vi "Driving.vi"(11 "input cluster":T2) -> (3 "Motor Info Cluster":T1)   [LabVIEW 2015]
uses:
  Joystick/ControlsToCommands.ctl
  References/Refnums.vi
panel:
  in  "Motor Values and Errors":T1
  out "Boolean":bool
  in  "valS":bool
  in  "PWM 5":dbl min=-1.0 max=1.0 step=1.0
  in  "PWM 4":dbl min=-1.0 max=1.0 step=1.0
  in  "PWM 3":dbl min=-1.0 max=1.0 step=1.0
  in  "PWM 2":dbl min=-1.0 max=1.0 step=1.0
  in  "PWM 1":dbl min=-1.0 max=1.0 step=1.0
  in  "PWM 0":dbl min=-1.0 max=1.0 step=1.0
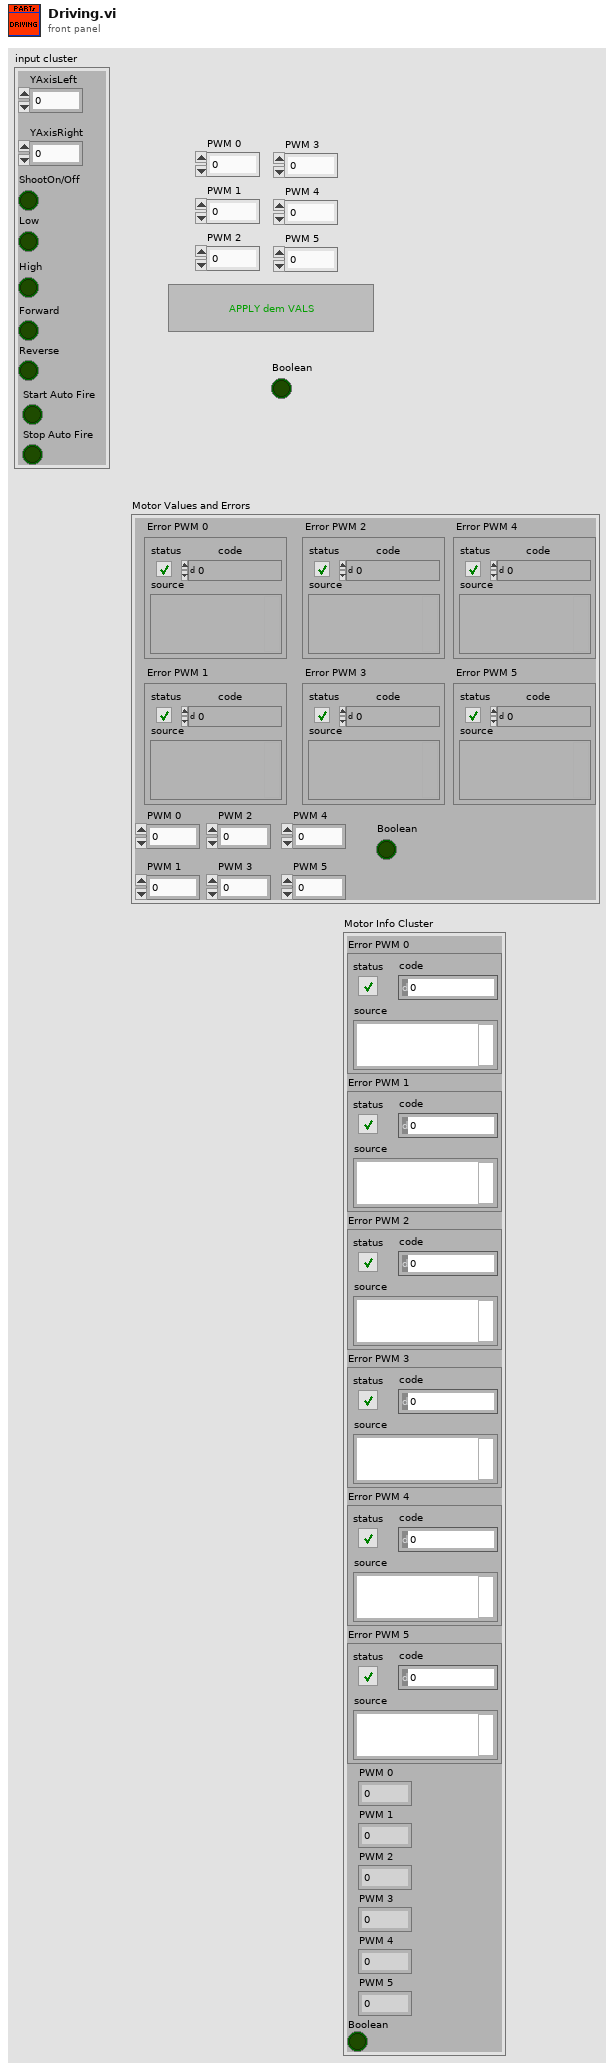
[diagram p1: front panel]
types:
  T1 = cluster{"Error PWM 0":errorcluster, "Error PWM 1":errorcluster, "Error PWM 2":errorcluster, "Error PWM 3":errorcluster, "Error PWM 4":errorcluster, "Error PWM 5":errorcluster, "PWM 0":dbl, "PWM 1":dbl, "PWM 2":dbl, "PWM 3":dbl, "PWM 4":dbl, "PWM 5":dbl, "Boolean":bool}
  T2 = typedef "ControlsToCommands.ctl" = cluster{"YAxisLeft":dbl, "YAxisRight":dbl, "ShootOn/Off":bool, "Low":bool, "High":bool, "Forward":bool, "Reverse":bool, "Start Auto Fire":bool, "Stop Auto Fire":bool}
  T3 = typedef "WPI_MotorControlDeviceRef.ctl" = cluster{"DeviceStatus":errorcluster, "Type":T4, "PWM":cluster{"PWM Channel":T5, "DeadBand":T6}, "CAN":cluster{"Device Number":u8, "Control Mode":T7, "Semaphore":T8, "Max Vout":dbl, "TalonSRX Control Mode":T9}, "Invert":bool}
  T4 = typedef "WPI_MotorControlType.ctl" = enum16{"PWM", "CAN", "CANTalonSRX"}
  T5 = typedef "FPGA_DIOPWMChannel.ctl" = enum8{"PWM 0", "PWM 1", "PWM 2", "PWM 3", "PWM 4", "PWM 5", "PWM 6", "PWM 7", "PWM 8", "PWM 9", "PWM MXP 0", "PWM MXP 1", "PWM MXP 2", "PWM MXP 3", "PWM MXP 4", "PWM MXP 5", "PWM MXP 6", "PWM MXP 7", "PWM MXP 8", "PWM MXP 9", "Invalid"}
  T6 = typedef "WPI_PWMDeadband.ctl" = cluster{"Name":string, "maxPositivePwm":i32, "minPositivePwm":i32, "centerPwm":i32, "maxNegativePwm":i32, "minNegativePwm":i32, "angularRange":u16}
  T7 = typedef "WPI_CANJaguar_ControlMode.ctl" = enum8{"Percent VBus", "Current", "Speed", "Position", "Voltage"}
  T8 = typedef "Semaphore RefNum" = refnum<k1>
  T9 = typedef "WPI_CANTalonSRX_APIControlMode.ctl" = enum8{"Percent VBus", "Speed", "Position", "Slave", "Unchanged / Invalid", "Voltage Compensation", "Current", "Motion Profile"}
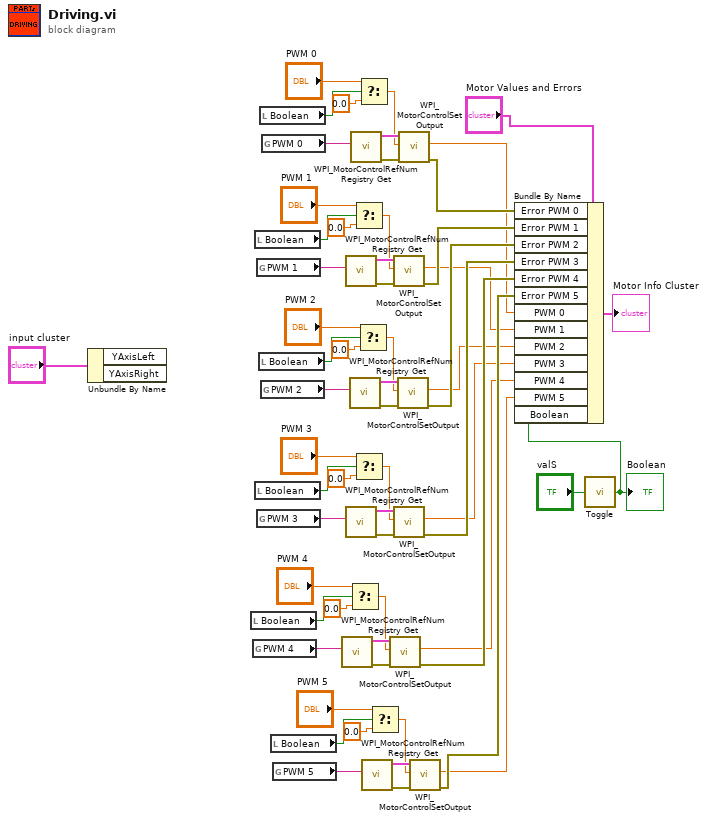
[diagram p0: block diagram]
diagram:
  n1 = Unbundle By Name("input cluster") -> ()  [unwired: 2 out]
  n2 = local read "Boolean"() -> (w28:bool)
  n3 = global read "Refnums.vi" "PWM 4"() -> (w56:string)
  n4 = local read "Boolean"() -> (w35:bool)
  n5 = local read "Boolean"() -> (w31:bool)
  n6 = global read "Refnums.vi" "PWM 1"() -> (w43:string)
  n7 = global read "Refnums.vi" "PWM 3"() -> (w55:string)
  n8 = local read "Boolean"() -> (w32:bool)
  n9 = local read "Boolean"() -> (w37:bool)
  n10 = global read "Refnums.vi" "PWM 2"() -> (w44:string)
  n11 = global read "Refnums.vi" "PWM 0"() -> (w49:string)
  n12 = local read "Boolean"() -> (w27:bool)
  n13 = global read "Refnums.vi" "PWM 5"() -> (w50:string)
  n14 = call <vilib>:"WPI_MotorControlRefNum Registry Get.vi"("refnum name"=w56) -> ("error out"=w58:errorcluster, "MotorControlDevRef"=w57:T3)  [unwired: 9 in]
  n15 = call <vilib>:"WPI_MotorControlRefNum Registry Get.vi"("refnum name"=w43) -> ("error out"=w41:errorcluster, "MotorControlDevRef"=w42:T3)  [unwired: 9 in]
  n16 = call <vilib>:"WPI_MotorControlRefNum Registry Get.vi"("refnum name"=w55) -> ("error out"=w53:errorcluster, "MotorControlDevRef"=w54:T3)  [unwired: 9 in]
  n17 = call <vilib>:"WPI_MotorControlRefNum Registry Get.vi"("refnum name"=w44) -> ("error out"=w46:errorcluster, "MotorControlDevRef"=w45:T3)  [unwired: 9 in]
  n18 = Select(t="PWM 4", s=w28, f=0.0) -> (s? t:f=w18:dbl)
  n19 = call <vilib>:"WPI_MotorControlRefNum Registry Get.vi"("refnum name"=w49) -> ("error out"=w47:errorcluster, "MotorControlDevRef"=w48:T3)  [unwired: 9 in]
  n20 = Select(t="PWM 1", s=w35, f=0.0) -> (s? t:f=w24:dbl)
  n21 = Select(t="PWM 3", s=w31, f=0.0) -> (s? t:f=w20:dbl)
  n22 = Select(t="PWM 2", s=w32, f=0.0) -> (s? t:f=w22:dbl)
  n23 = Select(t="PWM 0", s=w37, f=0.0) -> (s? t:f=w36:dbl)
  n24 = call <vilib>:"WPI_MotorControlRefNum Registry Get.vi"("refnum name"=w50) -> ("error out"=w52:errorcluster, "MotorControlDevRef"=w51:T3)  [unwired: 9 in]
  n25 = Select(t="PWM 5", s=w27, f=0.0) -> (s? t:f=w16:dbl)
  n26 = call <vilib>:"WPI_MotorControlSetOutput.vi"("error in (no error)"=w58, "Output"=w18, "MotorControlDevRef"=w57) -> ("error out"=w10:errorcluster, "Motor Output"=w5:dbl)  [unwired: 6 in, 1 out]
  n27 = call <vilib>:"WPI_MotorControlSetOutput.vi"("error in (no error)"=w41, "Output"=w24, "MotorControlDevRef"=w42) -> ("error out"=w13:errorcluster, "Motor Output"=w7:dbl)  [unwired: 6 in, 1 out]
  n28 = call <vilib>:"WPI_MotorControlSetOutput.vi"("error in (no error)"=w53, "Output"=w20, "MotorControlDevRef"=w54) -> ("error out"=w11:errorcluster, "Motor Output"=w6:dbl)  [unwired: 6 in, 1 out]
  n29 = call <vilib>:"WPI_MotorControlSetOutput.vi"("error in (no error)"=w46, "Output"=w22, "MotorControlDevRef"=w45) -> ("error out"=w12:errorcluster, "Motor Output"=w3:dbl)  [unwired: 6 in, 1 out]
  n30 = call <vilib>:"WPI_MotorControlSetOutput.vi"("error in (no error)"=w47, "Output"=w36, "MotorControlDevRef"=w48) -> ("error out"=w14:errorcluster, "Motor Output"=w8:dbl)  [unwired: 6 in, 1 out]
  n31 = call <vilib>:"WPI_MotorControlSetOutput.vi"("error in (no error)"=w52, "Output"=w16, "MotorControlDevRef"=w51) -> ("error out"=w9:errorcluster, "Motor Output"=w4:dbl)  [unwired: 6 in, 1 out]
  n32 = call "Toggle.vi"("Input"="valS") -> ("Output"=w2:bool)  [unwired: 4 in]
  "Boolean" <- w2
  n33 = Bundle By Name(cluster="Motor Values and Errors", "Error PWM 0"=w14, "Error PWM 1"=w13, "Error PWM 2"=w12, "Error PWM 3"=w11, "Error PWM 4"=w10, "Error PWM 5"=w9, "PWM 0"=w8, "PWM 1"=w7, "PWM 2"=w3, "PWM 3"=w6, "PWM 4"=w5, "PWM 5"=w4, "Boolean"=w2) -> (→"Motor Info Cluster":T1)
